vi "Compile Frames.vi"(8 "error in (no error)":errorcluster, 9 "Array in":cluster{"Type":T3, "Child Refs":T1[]}[](array[cluster]) {"Child Refs" format="%.0x"}, 10 "cluster":T9, 11 "Refnum in":refnum<k21>) -> (0 "error out":errorcluster, 1 "Array 3":T1[](array[typedef]) format="%.0x", 2 "Array 4":T1[](array[typedef]) format="%.0x", 3 "Array out":T2[](array[typedef]) {"Protection Configurations"."CRC Channels"."Data Type" items=["Signed", "Unsigned", "IEEE Float"]})   [LabVIEW 2015, in "Protection and Rolling Counter Addon System Explorer.lvlib"]
uses:
  Protection and Rolling Counter Addon System Explorer.lvlib
  Shared/Types/Exported Frame Type.ctl
  <vilib>/NI Veristand/Custom Device API/Custom Device Item Ref.ctl
  Shared/Types/Exported Frame Settings.ctl
  Shared/Types/Exported Protection Settings.ctl
  Shared/Types/Protection Type.ctl
  Shared/Types/InputChannelConfiguration.ctl
  Shared/Types/Exported Counter Settings.ctl
  Shared/Types/Event Trigger Type.ctl
  <vilib>/NI Veristand/Custom Device Tools/Custom Device Utility Library/NI VeriStand - Search for All Items by GUID.vi
  Shared/Protection and Rolling Counter Addon Shared.lvlib
  <vilib>/NI VeriStand/Custom Device API/Custom Device API.lvlib
  <resource>/objmgr/xnet.rc
  <vilib>/NI VeriStand/Custom Device Tools/Custom Device Utility Library/Custom Device Utility Library.lvlib
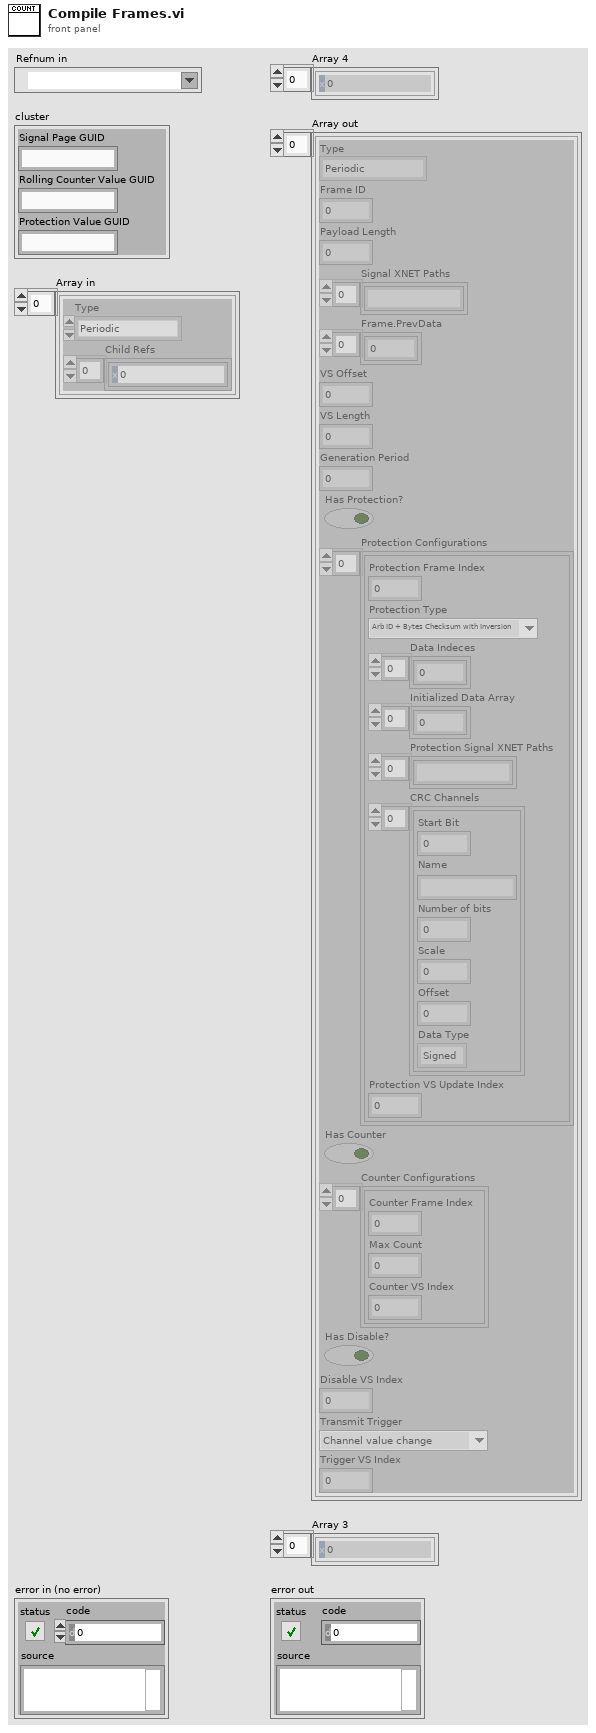
[diagram p1: front panel]
types:
  T1 = typedef "Custom Device API.lvlib/Custom Device Item Ref.ctl" = u64
  T2 = typedef "Protection and Rolling Counter Addon Shared.lvlib/Exported Frame Settings.ctl" = cluster{"Type":T3, "Frame ID":u32, "Payload Length":u32, "Signal XNET Paths":string[], "Frame.PrevData":dbl[], "VS Offset":i32, "VS Length":i32, "Generation Period":u32, "Has Protection?":bool, "Protection Configurations":T4[], "Has Counter":bool, "Counter Configurations":T7[], "Has Disable?":bool, "Disable VS Index":i32, "Transmit Trigger":T8, "Trigger VS Index":i32}
  T3 = typedef "Protection and Rolling Counter Addon Shared.lvlib/Exported Frame Type.ctl" = enum16{"Periodic", "Event", "Periodic/Event"}
  T4 = typedef "Protection and Rolling Counter Addon Shared.lvlib/Exported Protection Settings.ctl" = cluster{"Protection Frame Index":i32, "Protection Type":T5, "Data Indeces":i32[], "Initialized Data Array":dbl[], "Protection Signal XNET Paths":string[], "CRC Channels":T6[], "Protection VS Update Index":i32}
  T5 = typedef "Protection and Rolling Counter Addon Shared.lvlib/Protection Type.ctl" = enum16{"Arb ID + Bytes Checksum with Inversion", "Arb ID + Bytes CRC with Inversion", "Reversed Raw Signal Checksum with Inversion"}
  T6 = typedef "Protection and Rolling Counter Addon Shared.lvlib/InputChannelConfiguration.ctl" = cluster{"Start Bit":i32, "Name":string, "Number of bits":i32, "Scale":dbl, "Offset":dbl, "Data Type":u32}
  T7 = typedef "Protection and Rolling Counter Addon Shared.lvlib/Exported Counter Settings.ctl" = cluster{"Counter Frame Index":i32, "Max Count":dbl, "Counter VS Index":i32}
  T8 = typedef "Protection and Rolling Counter Addon Shared.lvlib/Event Trigger Type.ctl" = enum16{"Channel value change", "Trigger channel (not zero)", "Channel value change or trigger channel (not zero)", "Trigger channel (any value change)", "Channel value change or trigger channel (any value change)"}
  T9 = cluster{"Signal Page GUID":string, "Rolling Counter Value GUID":string, "Protection Value GUID":string}
  T10 = typedef "Custom Device API.lvlib/Custom Device Item Info.ctl" = cluster{"Name":string, "Is Channel":bool, "GUID":string, "Is Waveform":bool}
  T11 = typedef "Protection and Rolling Counter Addon System Explorer.lvlib/Frame Settings.ctl" = cluster{"ID":u32, "Disable Transmission":bool, "Disable Transmission Ref":T1, "Transmit Trigger":T8, "Transmit Trigger Ref":T1}
  T12 = typedef "Protection and Rolling Counter Addon System Explorer.lvlib/Protection Signal Settings.ctl" = cluster{"Input Channels":T13[], "Protection Type":T5}
  T13 = typedef "Protection and Rolling Counter Addon System Explorer.lvlib/Protection Signal Linked Channels.ctl" = cluster{"Node Ref":T1}
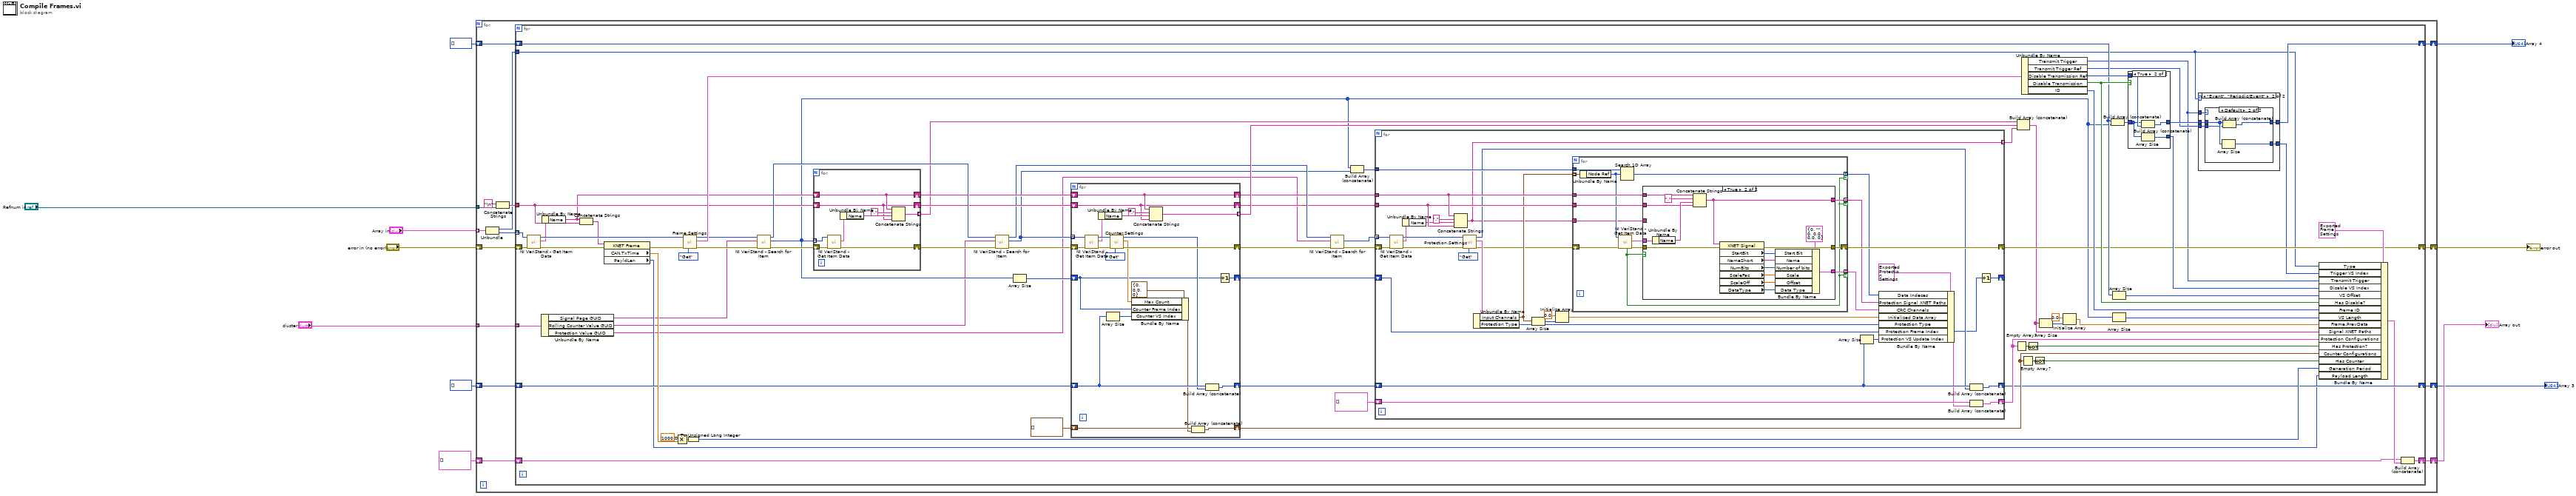
[diagram p0: block diagram]
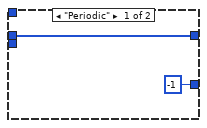
[diagram p2: hidden frame]
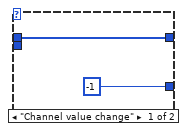
[diagram p3: hidden frame]
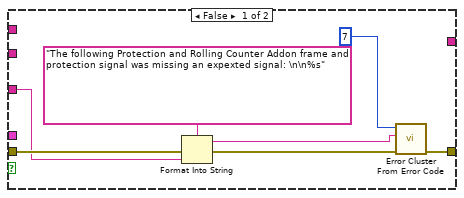
[diagram p4: hidden frame]
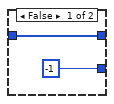
[diagram p5: hidden frame]
diagram:
  n1 = for {
    tunnel: "Refnum in" -> [w26]
    shift-right: [w21] -> w4
    shift-left: "error in (no error)" -> [w15]
    shift-right: [w20] -> w5
    shift-left: T2[] [] -> [w19]
    shift-right: [w23] -> w2
    shift-left: T1[] [] -> [w18]
    shift-right: [w22] -> w3
    shift-left: T1[] [] -> [w17]
    tunnel: "cluster" -> [w16]
    tunnel: "Array in" -> [w14] mode=indexing
    n2 = Unbundle(w14) -> ("Type"=w12:T3, "Child Refs"=w13:T1[])
    n3 = Concatenate Strings("\n", w26) -> (w24:string)
    n4 = for {
      tunnel: w13 -> [w81] mode=indexing
      shift-right: [w48] -> w21
      shift-left: w15 -> [w82]
      shift-right: [w93] -> w23
      shift-left: w18 -> [w91]
      tunnel: w24 -> [w64]
      shift-right: [w42] -> w22
      shift-left: w17 -> [w70]
      shift-right: [w33] -> w20
      shift-left: w19 -> [w32]
      tunnel: w12 -> [w31]
      tunnel: w16 -> [w30]
      n5 = call <vilib>:"NI VeriStand - Get Item Data.vi"("error in (no error)"=w82, "Item Ref in"=w81) -> ("error out"=w77:errorcluster, "Item Info"=w79:T10, "Item Ref out"=w80:T1)  [unwired: 6 in, 1 out]
      n6 = Unbundle By Name(w30) -> ("Signal Page GUID"=w29:string, "Rolling Counter Value GUID"=w28:string, "Protection Value GUID"=w27:string)
      n7 = Unbundle By Name(w79) -> ("Name"=w63:string)
      n8 = Concatenate Strings(w63, w64) -> (w78:string)
      n9 = property class="XNET Frame"(reference=w78, error in=w77) -> (error out=w76:errorcluster, "CAN.TxTime"=w74:dbl, "PayldLen"=w38:u32)  [unwired: 1 out]
      n10 = Multiply(x=1000.0 ("y"), y=w74) -> (x*y=w75:dbl)
      n11 = call "Frame.Settings.vi"("Action"=enum8{"Get", "Set"}."Get", "error in (no error)"=w76, "Item Ref in"=w80) -> ("error out"=w99:errorcluster, "Frame.Settings"=w100:T11, "Item Ref out"=w97:T1)  [unwired: 6 in]
      n12 = To Unsigned Long Integer(number=w75) -> (unsigned 32bit integer=w72:u32)
      n13 = call-poly <vilib>:"NI VeriStand - Search for Item.vi"("error in"=w99, "Item GUID"=w29, "Section Ref in"=w97) -> ("error out"=w66:errorcluster, "Item Refs"=w40:T1[], "Section Ref out"=w69:T1)  [unwired: 5 in, 1 out]
      n14 = for {
        tunnel: w40 -> [w194] mode=indexing
        shift-right: [w188] -> w65
        shift-left: w66 -> [w193]
        tunnel: [w190] -> w60 mode=indexing
        shift-right: [w187] -> w62
        shift-left: w63 -> [w187]
        shift-right: [w186] -> w61
        shift-left: w64 -> [w186]
        n15 = call <vilib>:"NI VeriStand - Get Item Data.vi"("error in (no error)"=w193, "Item Ref in"=w194) -> ("error out"=w188:errorcluster, "Item Info"=w189:T10)  [unwired: 6 in, 2 out]
        n16 = Unbundle By Name(w189) -> ("Name"=w191:string)
        n17 = Concatenate Strings(w187, "." ("string"), w191, w186) -> (w190:string)
      }
      n18 = call-poly <vilib>:"NI VeriStand - Search for Item.vi"("error in"=w65, "Item GUID"=w28, "Section Ref in"=w69) -> ("error out"=w68:errorcluster, "Item Refs"=w39:T1[], "Section Ref out"=w57:T1)  [unwired: 5 in, 1 out]
      n19 = Array Size(array=w40) -> (size(s)=w67:i32)
      n20 = for {
        tunnel: w39 -> [w217] mode=indexing
        shift-right: [w211] -> w58
        shift-left: w68 -> [w216]
        shift-right: [w213] -> w83
        shift-left: T7[] [] -> [w212]
        tunnel: [w208] -> w59 mode=indexing
        shift-right: [w205] -> w43
        shift-left: w70 -> [w206]
        shift-right: [w198] -> w53
        shift-left: w67 -> [w199]
        shift-right: [w197] -> w51
        shift-left: w62 -> [w197]
        shift-right: [w196] -> w52
        shift-left: w61 -> [w196]
        n21 = call <vilib>:"NI VeriStand - Get Item Data.vi"("error in (no error)"=w216, "Item Ref in"=w217) -> ("error out"=w214:errorcluster, "Item Info"=w207:T10, "Item Ref out"=w215:T1)  [unwired: 6 in, 1 out]
        n22 = Unbundle By Name(w207) -> ("Name"=w209:string)
        n23 = Array Size(array=w206) -> (size(s)=w200:i32)
        n24 = call "Counter.Settings.vi"("Action"=enum8{"Get", "Set"}."Get", "error in"=w214, "Parent Ref"=w215) -> ("error out"=w211:errorcluster, "Max Count"=w204:dbl, "Parent Ref Out"=w201:T1)  [unwired: 6 in]
        n25 = Bundle By Name(cluster=T7 {"Counter Frame Index"=0, "Max Count"=0.0, "Counter VS Index"=0} ("Cluster"), "Max Count"=w204, "Counter Frame Index"=w199, "Counter VS Index"=w200) -> (w203:T7)
        n26 = Concatenate Strings(w197, "." ("string"), w209, w196) -> (w208:string)
        n27 = Build Array (concatenate)(w212, w203) -> (w213:T7[])
        n28 = Build Array (concatenate)(w206, w201) -> (w205:T1[])
        n29 = Increment(x=w199) -> (x+1=w198:i32)
      }
      n30 = call-poly <vilib>:"NI VeriStand - Search for Item.vi"("error in"=w58, "Item GUID"=w27, "Section Ref in"=w57) -> ("error out"=w56:errorcluster, "Item Refs"=w55:T1[])  [unwired: 5 in, 2 out]
      n31 = Build Array (concatenate)(w40, w39) -> (w41:T1[])
      n32 = for {
        tunnel: w55 -> [w148] mode=indexing
        shift-right: [w141] -> w48
        shift-left: w56 -> [w147]
        shift-right: [w142] -> w49
        shift-left: T4[] [] -> [w144]
        tunnel: w41 -> [w143]
        tunnel: w51 -> [w139]
        tunnel: [w117] -> w50 mode=indexing
        shift-right: [w135] -> w42
        shift-left: w43 -> [w136]
        shift-right: [w119] -> _
        shift-left: w53 -> [w120]
        tunnel: w52 -> [w138]
        n33 = call <vilib>:"NI VeriStand - Get Item Data.vi"("error in (no error)"=w147, "Item Ref in"=w148) -> ("error out"=w145:errorcluster, "Item Info"=w137:T10, "Item Ref out"=w146:T1)  [unwired: 6 in, 1 out]
        n34 = Unbundle By Name(w137) -> ("Name"=w118:string)
        n35 = Concatenate Strings(w139, "." ("string"), w118, w138) -> (w117:string)
        n36 = call "Protection.Settings.vi"("Action"=enum8{"Get", "Set"}."Get", "error in"=w145, "Parent Ref"=w146) -> ("error out"=w125:errorcluster, "Selected Channels"=w134:T12, "Parent Ref Out"=w121:T1)  [unwired: 6 in]
        n37 = Unbundle By Name(w134) -> ("Input Channels"=w131:T13[], "Protection Type"=w133:T5)
        n38 = Array Size(array=w131) -> (size(s)=w130:i32)
        n39 = Initialize Array(0.0 ("element"), w130) -> (w128:dbl[])
        n40 = for {
          tunnel: w143 -> [w152]
          tunnel: w131 -> [w162] mode=indexing
          tunnel: [w161] -> w132 mode=indexing if=w150
          shift-right: [w155] -> w141
          shift-left: w125 -> [w160]
          tunnel: w139 -> [w158]
          tunnel: w138 -> [w157]
          tunnel: [w153] -> w124 mode=indexing if=w150
          tunnel: [w154] -> w126 mode=indexing if=w150
          tunnel: w117 -> [w149]
          n41 = Unbundle By Name(w162) -> ("Node Ref"=w151:T1)
          n42 = call <vilib>:"NI VeriStand - Get Item Data.vi"("error in (no error)"=w160, "Item Ref in"=w151) -> ("error out"=w156:errorcluster, "Item Info"=w159:T10, "Found"=w150:bool)  [unwired: 6 in, 1 out]
          n43 = Search 1D Array(1D array=w152, element=w151) -> (index of element=w161:i32)  [unwired: 1 in]
          n44 = case shown="True" w150 {
            tunnel: w159 -> [_ w185]
            tunnel: w158 -> [_ w182]
            tunnel: w157 -> [_ w181]
            tunnel: w156 -> [w167 w180]
            tunnel: [w169 w179] -> w155
            tunnel: [_ w171] -> w154
            tunnel: [_ w170] -> w153
            tunnel: w149 -> [w164 _]
            frame False {
              n45 = Format Into String(format string="The following Protection and Rolling Counter Addon frame and protection signal was missing an expexted signal: \n\n%s" ("error message (\"\")"), error in=w167, w164) -> (resulting string=w163:string, error out=w166:errorcluster)  [unwired: 1 in]
              n46 = call <vilib>:"Error Cluster From Error Code.vi"("error in (no error)"=w166, "error message (\"\")"=w163, "error code (0)"=7) -> ("error out"=w169:errorcluster)  [unwired: 6 in]
            }
            frame True {
              n47 = Unbundle By Name(w185) -> ("Name"=w183:string)
              n48 = Concatenate Strings(w182, "." ("string"), w183, w181) -> (w170:string)
              n49 = property class="XNET Signal"(reference=w170, error in=w180) -> (error out=w179:errorcluster, "StartBit"=w172:u32, "NameShort"=w173:string, "NumBits"=w174:u32, "ScaleFac"=w175:dbl, "ScaleOff"=w176:dbl, "DataType"=w177:u32)  [unwired: 1 out]
              n50 = Bundle By Name(cluster=T6 {"Start Bit"=0, "Name"="", "Number of bits"=0, "Scale"=0.0, "Offset"=0.0, "Data Type"=0} ("MonitoredChannelSettings"), "Start Bit"=w172, "Name"=w173, "Number of bits"=w174, "Scale"=w175, "Offset"=w176, "Data Type"=w177) -> (w171:T6)
            }
          }
        }
        n51 = Array Size(array=w136) -> (size(s)=w122:i32)
        n52 = Bundle By Name(cluster=T4 {"Protection Frame Index"=0, "Protection Type"=enum."Arb ID + Bytes Checksum with Inversion", "Data Indeces"=[], "Initialized Data Array"=[], "Protection Signal XNET Paths"=[], "CRC Channels"=[], "Protection VS Update Index"=0} ("Cluster"), "Data Indeces"=w132, "Protection Signal XNET Paths"=w124, "CRC Channels"=w126, "Initialized Data Array"=w128, "Protection Type"=w133, "Protection Frame Index"=w120, "Protection VS Update Index"=w122) -> (w127:T4)
        n53 = Build Array (concatenate)(w136, w121) -> (w135:T1[])
        n54 = Build Array (concatenate)(w144, w127) -> (w142:T4[])
        n55 = Increment(x=w120) -> (x+1=w119:i32)
      }
      n56 = Empty Array?(array=w49) -> (empty?=w85:bool)
      n57 = Build Array (concatenate)(w60, w59, w50) -> (w47:string[])
      n58 = Unbundle By Name(w100) -> ("Transmit Trigger"=w36:T8, "Transmit Trigger Ref"=w37:T1, "Disable Transmission Ref"=w95:T1, "Disable Transmission"=w96:bool, "ID"=w98:u32)
      n59 = Empty Array?(array=w83) -> (empty?=w87:bool)
      n60 = Not(x=w85) -> (.not. x?=w84:bool)
      n61 = Not(x=w87) -> (.not. x?=w86:bool)
      n62 = Array Size(array=w47) -> (size(s)=w45:i32)
      n63 = Initialize Array(0.0 ("element"), w45) -> (w44:dbl[])
      n64 = Build Array (concatenate)(w91, w40) -> (w92:T1[])
      n65 = Array Size(array=w91) -> (size(s)=w90:i32)
      n66 = Array Size(array=w40) -> (size(s)=w71:i32)
      n67 = case shown="True" w96 {
        tunnel: w92 -> [w219 w221]
        tunnel: [w219 w223] -> w94
        tunnel: w95 -> [_ w222]
        tunnel: [-1 w220] -> w89
        frame False {
        }
        frame True {
          n68 = Build Array (concatenate)(w221, w222) -> (w223:T1[])
          n69 = Array Size(array=w221) -> (size(s)=w220:i32)
        }
      }
      n70 = case shown="\"Event\", \"Periodic/Event\"" w31 {
        tunnel: w94 -> [w104 w109]
        tunnel: [w104 w108] -> w93
        tunnel: w37 -> [_ w107]
        tunnel: w36 -> [_ w106]
        tunnel: [-1 w105] -> w35
        frame "Periodic" {
        }
        frame "Event", "Periodic/Event" {
          n71 = case shown="Default" w106 {
            tunnel: w109 -> [w111 w114]
            tunnel: [w111 w115] -> w108
            tunnel: [-1 w113] -> w105
            tunnel: w107 -> [_ w112]
            frame "Channel value change" {
            }
            frame Default {
              n72 = Array Size(array=w114) -> (size(s)=w113:i32)
              n73 = Build Array (concatenate)(w114, w112) -> (w115:T1[])
            }
          }
        }
      }
      n74 = Bundle By Name(cluster=T2 {"Type"=enum."Periodic", "Frame ID"=0, "Payload Length"=0, "Signal XNET Paths"=[], "Frame.PrevData"=[], "VS Offset"=0, "VS Length"=0, "Generation Period"=0, "Has Protection?"=FALSE, "Protection Configurations"=[], "Has Counter"=FALSE, "Counter Configurations"=[], "Has Disable?"=FALSE, "Disable VS Index"=0, "Transmit Trigger"=enum."Channel value change", "Trigger VS Index"=0} ("Frame Settings"), "Type"=w31, "Trigger VS Index"=w35, "Transmit Trigger"=w36, "Disable VS Index"=w89, "VS Offset"=w90, "Has Disable?"=w96, "Frame ID"=w98, "VS Length"=w71, "Frame.PrevData"=w44, "Signal XNET Paths"=w47, "Protection Configurations"=w49, "Has Protection?"=w84, "Counter Configurations"=w83, "Has Counter"=w86, "Generation Period"=w72, "Payload Length"=w38) -> (w34:T2)
      n75 = Build Array (concatenate)(w32, w34) -> (w33:T2[])
    }
  }
  "Array out" <- w5
  "error out" <- w4
  "Array 3" <- w3
  "Array 4" <- w2
